vi "generate name.vi"(1 "varient in":variant) -> (0 "name":string)   [LabVIEW 2020, in "Publisher Subscriber.lvlib"]
uses:
  Publisher Subscriber.lvlib
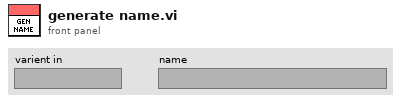
[diagram p1: front panel]
types:
  T1 = enum8{"<Null>", "I8", "I16", "I32", "I64", "U8", "U16", "U32", "U64", "SGL", "DBL", "EXT", "CSG", "CDB", "CXT", "0x0F", "0x10", "0x11", "0x12", "0x13", "0x14", "Enum U8", "Enum U16", "Enum U32", "Enum U64", "SGL PQ", "DBL PQ", "EXT PQ", "CSG PQ", "CDB PQ", "CXT PQ", "0x1F", "0x20", "Boolean", "0x22", "0x23", "0x24", "0x25", "0x26", "0x27", "0x28", "0x29", "0x2A", "0x2B", "0x2C", "0x2D", "0x2E", "0x2F", "String", "0x31", "Path", "Pict", "0x34", "0x35", "0x36", "DAQ", "0x38", "0x39", "0x3A", "0x3B", "0x3C", "0x3D", "0x3E", "0x3F", "Array", "0x41", "0x42", "0x43", "0x44", "0x45", "0x46", "0x47", "0x48", "0x49", "0x4A", "0x4B", "0x4C", "0x4D", "0x4E", "0x4F", "Cluster", "0x51", "0x52", "Variant", "Waveform", "0x55", "0x56", "0x57", "0x58", "0x59", "0x5A", "0x5B", "0x5C", "0x5D", "0x5E", "Fixed Point", "0x60", "0x61", "0x62", "0x63", "0x64", "0x65", "0x66", "0x67", "0x68", "0x69", "0x6A", "0x6B", "0x6C", "0x6D", "0x6E", "0x6F", "Refnum", "0x71", "0x72", "Set Collection", "Map Collection"}
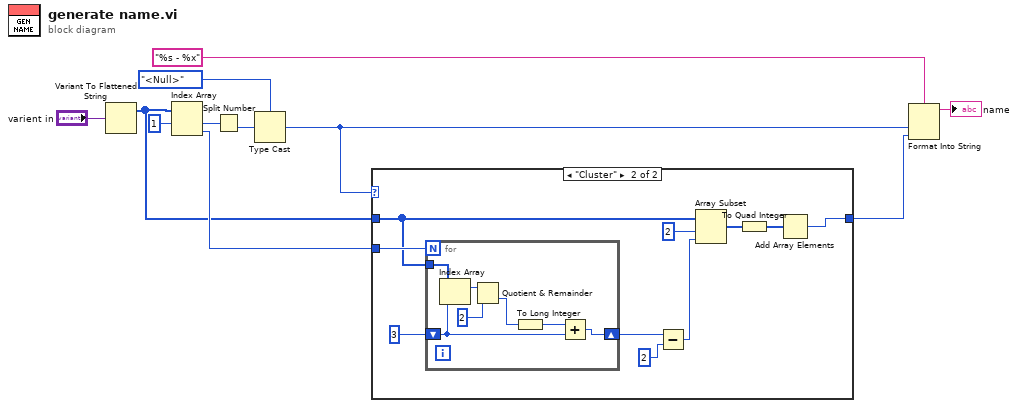
[diagram p0: block diagram]
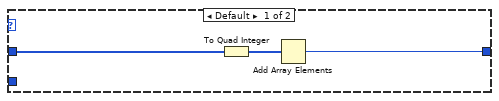
[diagram p2: hidden frame]
diagram:
  n1 = Variant To Flattened String(Variant="varient in") -> (1:w2:i16[])  [unwired: 1 out]
  n2 = Index Array(array=w2, index #1=1 ("index")) -> (element #1=w11:i16, element #2=w3:i16)  [unwired: 1 in]
  n3 = Split Number(x=w11) -> (lo(x)=w7:u8)  [unwired: 1 out]
  n4 = Type Cast(type=T1."<Null>", x=w7) -> (*(type *) &x=w4:T1)
  n5 = case shown="\"Cluster\"" w4 {
    tunnel: w3 -> [_ w19]
    tunnel: w2 -> [w13 w18]
    tunnel: [w12 w15] -> w1
    frame Default {
      n6 = To Quad Integer(1:w13) -> (0:w14:i64[])
      n7 = Add Array Elements(numeric array=w14) -> (sum=w12:i64)
    }
    frame "Cluster" {
      n8 = for {
        N: w19 -> [_]
        shift-right: [w30] -> w22
        shift-left: 3 -> [w29]
        tunnel: w18 -> [w31]
        n9 = Index Array(array=w31, index=w29) -> (element=w27:i16)
        n10 = Quotient & Remainder(x=w27, y=i16 2) -> (floor(x/y)=w28:i16)  [unwired: 1 out]
        n11 = To Long Integer(number=w28) -> (32bit integer=w25:i32)
        n12 = Add(x=w25, y=w29) -> (x+y=w30:i32)
      }
      n13 = Subtract(x=w22, y=2) -> (x-y=w21:i32)
      n14 = Array Subset(array=w18, index=2, length=w21) -> (w16:i16[])
      n15 = To Quad Integer(1:w16) -> (0:w17:i64[])
      n16 = Add Array Elements(numeric array=w17) -> (sum=w15:i64)
    }
  }
  n17 = Format Into String(format string="%s - %x", w4, w1) -> (resulting string=→"name":string)  [unwired: 2 in, 1 out]
